vi "AC Transport Configure.vi"(0 "6221 Address":string="13", 1 "SR860 Ch1 Address":string="4", 2 "Ch1 Enable":bool=TRUE, 3 "SR860 Ch2 Address":string="5", 4 "Ch2 Enable":bool=TRUE, 5 "Current Amplitude":string="1e-4", 7 "Frequency":string="17.32", 9 "Filter BW":T2(ring)=enum."100ms", 11 "Buffer Size (kB)":i32=2, 12 "Ch1 Harmonic":T1(ring), 13 "Ch2 Harmonic":T1(ring), 14 "Rate decimation":i32=2) -> (8 "Error 6221":errorcluster, 10 "Error SR860 Ch1":errorcluster, 15 "Error SR860 Ch2":errorcluster)   [LabVIEW 2020]
panel:
  in  "INIT 6221":bool=TRUE
  in  "Buffer Data":enum16{"X", "XY", "RT", "XYRT"}(ring)=enum."RT"
  out "SR860 Commands":string="*RST;\nIVMD VOLTAGE;\nISRC A-B;\nICPL AC;\nIGND GROund;\nSYNC OFF;\nOFSL 3;\nOFLT 10;\nRSRC EXT;\nRTRG NEGttl;\nREFZ 1Meg;\nHARM 1;\nARNG;\nASCL;\nAPHS;\nCAPTURELEN 2;\nCAPTURECFG 2;\nCAPTURERATE 2;\n"
  in  "TRIG Wave":bool
  out "6221 Commands":string="*RST\nTRIG:OLIN 4\nOUTP:LTEarth ON\nSOUR:WAVE:AMPL 1e-4\nSOUR:WAVE:FREQ 17.32\nSOUR:WAVE:FUNC SIN\nSOUR:WAVE:OFFS 0\nSOUR:WAVE:PMAR:STAT ON\nSOUR:WAVE:PMAR:OLIN 2\nSOUR:WAVE:RANG BEST\nSOUR:CURR:COMP 25\nSOUR:WAVE:ARM"
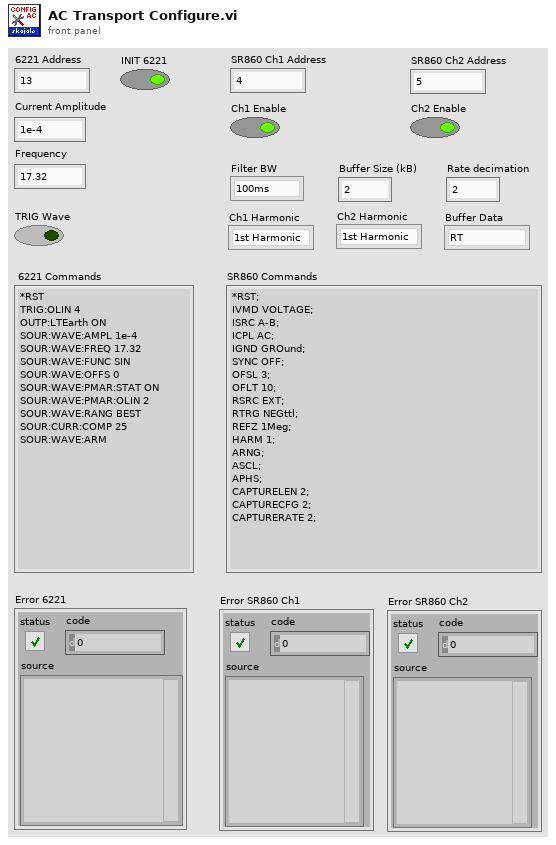
[diagram p1: front panel]
types:
  T1 = enum16{"1st Harmonic", "2nd Harmonic", "3rd Harmonic"}
  T2 = enum16{"1us", "3us", "10us", "30us", "100us", "300us", "1ms", "3ms", "10ms", "30ms", "100ms", "300ms", "1s"}
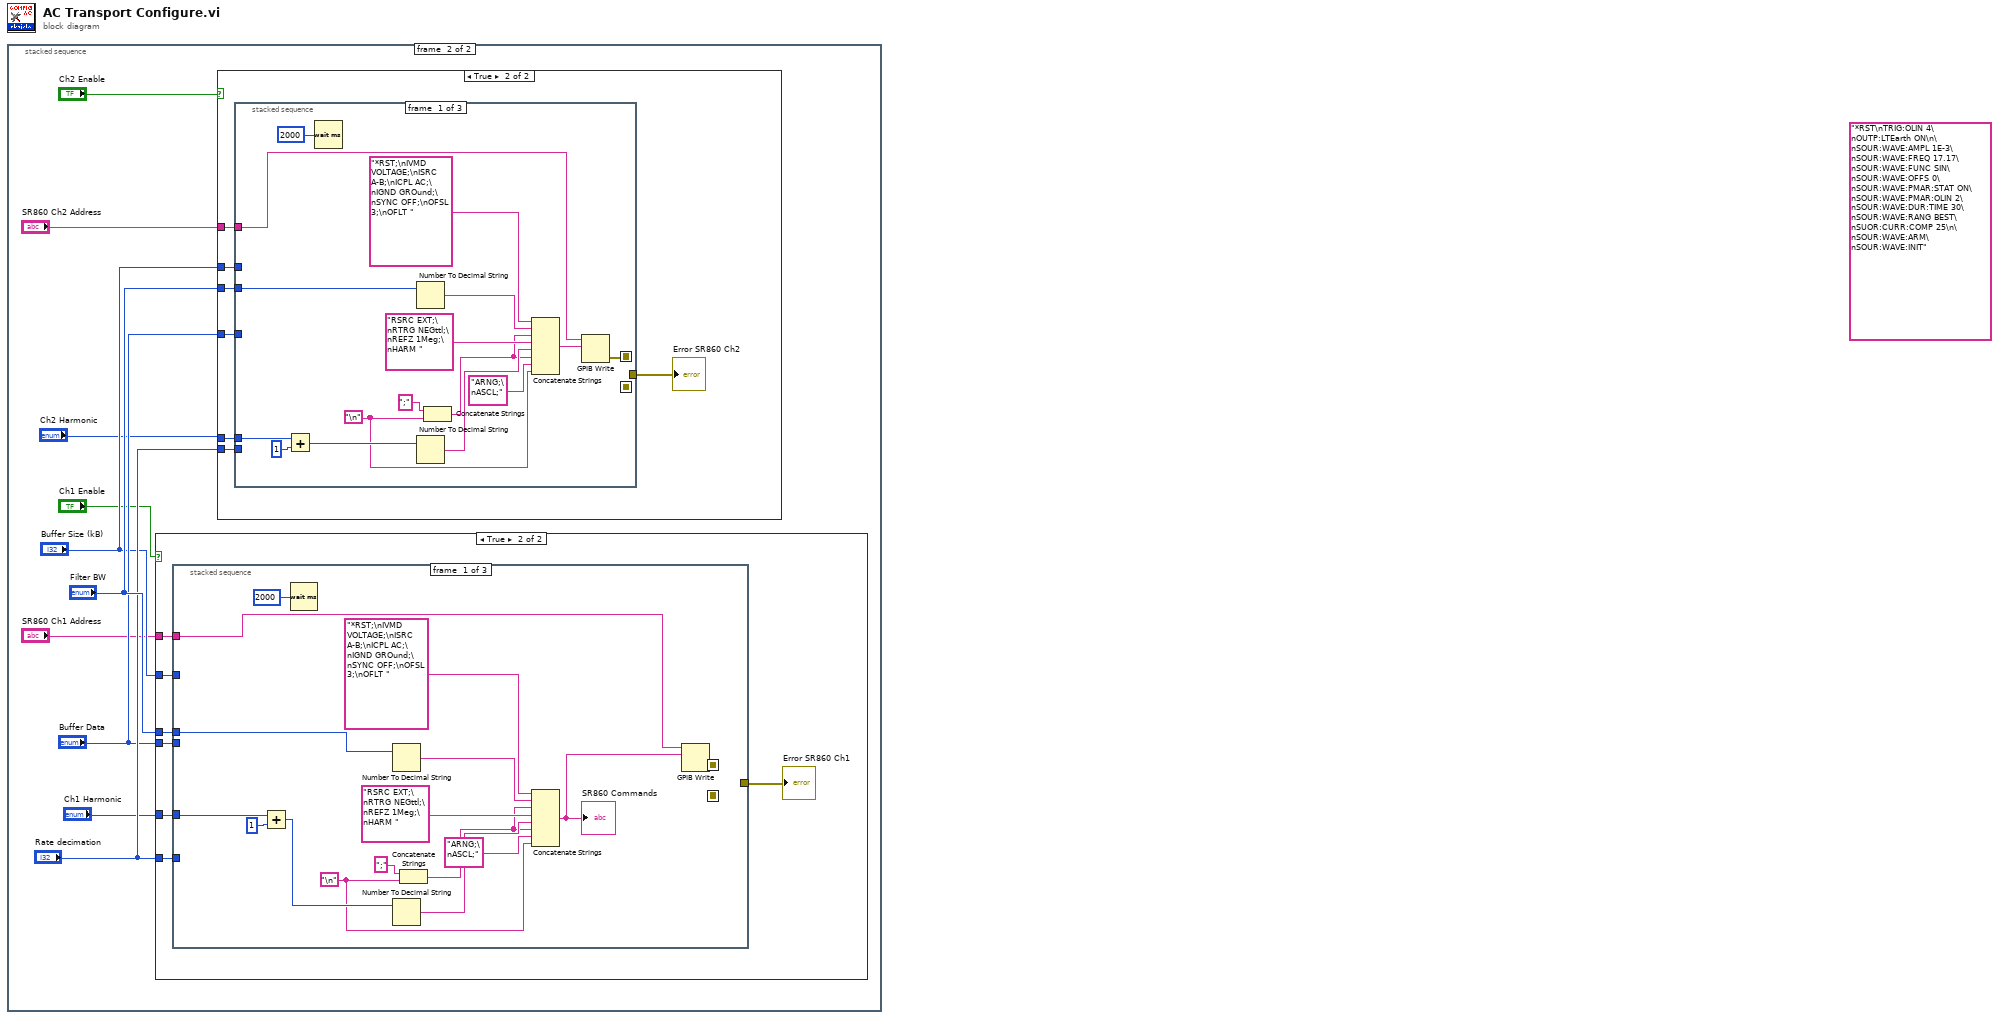
[diagram p0: block diagram]
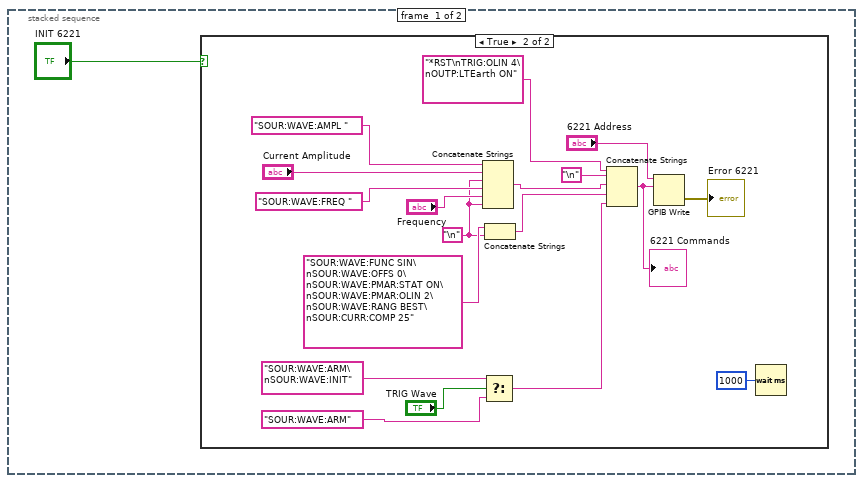
[diagram p2: hidden frame]
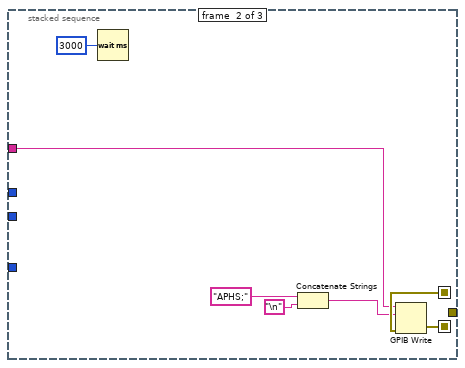
[diagram p5: hidden frame]
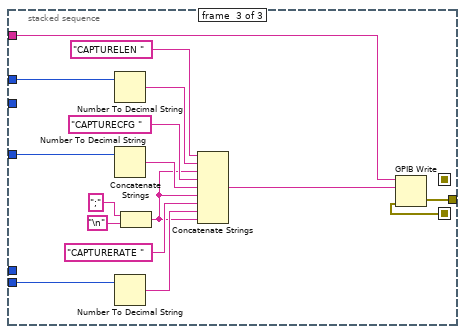
[diagram p6: hidden frame]
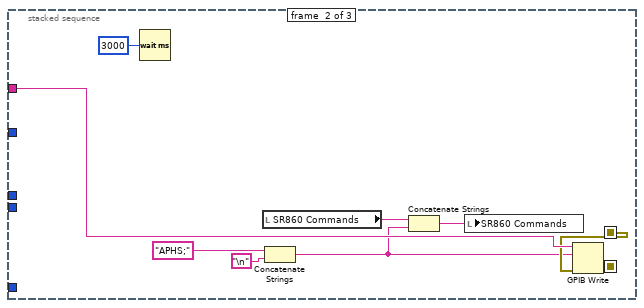
[diagram p8: hidden frame]
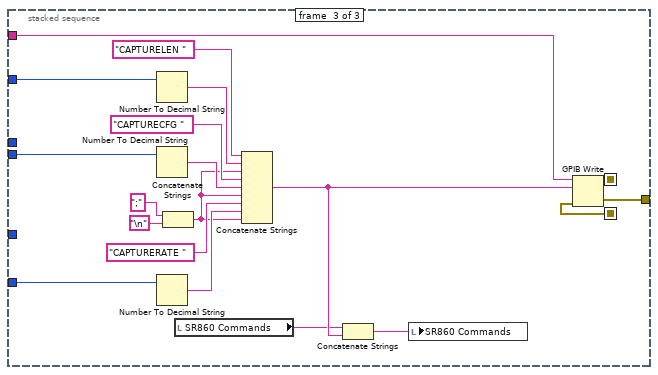
[diagram p9: hidden frame]
diagram:
  (unwired) "*RST\nTRIG:OLIN 4\nOUTP:LTEarth ON\n\nSOUR:WAVE:AMPL 1E-3\nSOUR:WAVE:FREQ 17.17\nSOUR:WAVE:FUNC SIN\nSOUR:WAVE:OFFS 0\nSOUR:WAVE:PMAR:STAT ON\nSOUR:WAVE:PMAR:OLIN 2\nSOUR:WAVE:DUR:TIME 30\nSOUR:WAVE:RANG BEST\nSUOR:CURR:COMP 25\n\nSOUR:WAVE:ARM\nSOUR:WAVE:INIT" ("data")
  n1 = stacked-sequence {
    frame #0 {
      n2 = case shown="True" "INIT 6221" {
        frame False {
        }
        frame True {
          w4 = "\n"
          n3 = Concatenate Strings("SOUR:WAVE:AMPL ", "Current Amplitude", w4, "SOUR:WAVE:FREQ ", "Frequency", w4) -> (w14:string)
          n4 = Select(t="SOUR:WAVE:ARM\nSOUR:WAVE:INIT" ("string"), s="TRIG Wave", f="SOUR:WAVE:ARM" ("string")) -> (s? t:f=w10:string)
          n5 = Concatenate Strings("SOUR:WAVE:FUNC SIN\nSOUR:WAVE:OFFS 0\nSOUR:WAVE:PMAR:STAT ON\nSOUR:WAVE:PMAR:OLIN 2\nSOUR:WAVE:RANG BEST\nSOUR:CURR:COMP 25", w4) -> (w13:string)
          n6 = Concatenate Strings("*RST\nTRIG:OLIN 4\nOUTP:LTEarth ON", "\n", w14, w13, w10) -> (w12:string)
          "6221 Commands" <- w12
          n7 = GPIB Write(0:"6221 Address", 1:w12) -> (6:→"Error 6221":errorcluster)  [unwired: 3 in, 1 out]
          n8 = Wait (ms)(milliseconds to wait=u32 1000) -> ()  [unwired: 1 out]
        }
      }
    }
    frame #1 {
      n9 = case shown="True" "Ch1 Enable" {
        tunnel: "SR860 Ch1 Address" -> [_ w82]
        tunnel: "Rate decimation" -> [_ w80]
        tunnel: "Buffer Data" -> [_ w79]
        tunnel: "Buffer Size (kB)" -> [_ w78]
        tunnel: "Filter BW" -> [_ w77]
        tunnel: "Ch1 Harmonic" -> [_ w76]
        frame False {
        }
        frame True {
          n10 = stacked-sequence {
            seq-local: [w85 _ _] -> [_ w106 _]
            seq-local: [_ w105 _] -> [_ _ w116]
            tunnel: w82 -> [w86 w107 w114]
            tunnel: [_ _ w115] -> w81
            tunnel: w80 -> [_ _ w110]
            tunnel: w79 -> [_ _ w109]
            tunnel: w78 -> [_ _ w108]
            tunnel: w77 -> [w84 _ _]
            tunnel: w76 -> [w83 _ _]
            frame #0 {
              w89 = "\n"
              n11 = Add(x=w83, y=1) -> (x+y=w92:i32)
              n12 = Wait (ms)(milliseconds to wait=u32 2000) -> ()  [unwired: 1 out]
              n13 = Number To Decimal String(number=w84) -> (decimal integer string=w97:string)  [unwired: 1 in]
              n14 = Number To Decimal String(number=w92) -> (decimal integer string=w94:string)  [unwired: 1 in]
              n15 = Concatenate Strings(";" ("string"), w89) -> (w93:string)
              n16 = Concatenate Strings("*RST;\nIVMD VOLTAGE;\nISRC A-B;\nICPL AC;\nIGND GROund;\nSYNC OFF;\nOFSL 3;\nOFLT ", w97, w93, "RSRC EXT;\nRTRG NEGttl;\nREFZ 1Meg;\nHARM ", w94, w93, "ARNG;\nASCL;", w89) -> (w87:string)
              "SR860 Commands" <- w87
              n17 = GPIB Write(0:w86, 1:w87) -> (6:w85:errorcluster)  [unwired: 3 in, 1 out]
            }
            frame #1 {
              n18 = Wait (ms)(milliseconds to wait=u32 3000) -> ()  [unwired: 1 out]
              n19 = local read "SR860 Commands"() -> (w101:string)
              n20 = Concatenate Strings("APHS;", "\n") -> (w102:string)
              n21 = Concatenate Strings(w101, w102) -> (w100:string)
              n22 = local write "SR860 Commands"(w100) -> ()
              n23 = GPIB Write(0:w107, 1:w102, 3:w106) -> (6:w105:errorcluster)  [unwired: 2 in, 1 out]
            }
            frame #2 {
              n24 = Number To Decimal String(number=w108) -> (decimal integer string=w124:string)  [unwired: 1 in]
              n25 = Number To Decimal String(number=w109) -> (decimal integer string=w121:string)  [unwired: 1 in]
              n26 = Number To Decimal String(number=w110) -> (decimal integer string=w118:string)  [unwired: 1 in]
              n27 = Concatenate Strings(";" ("string"), "\n") -> (w117:string)
              n28 = local read "SR860 Commands"() -> (w111:string)
              n29 = Concatenate Strings("CAPTURELEN ", w124, w117, "CAPTURECFG ", w121, w117, "CAPTURERATE ", w118, w117) -> (w113:string)
              n30 = Concatenate Strings(w111, w113) -> (w112:string)
              n31 = local write "SR860 Commands"(w112) -> ()
              n32 = GPIB Write(0:w114, 1:w113, 3:w116) -> (6:w115:errorcluster)  [unwired: 2 in, 1 out]
            }
          }
          "Error SR860 Ch1" <- w81
        }
      }
      n33 = case shown="True" "Ch2 Enable" {
        tunnel: "Buffer Size (kB)" -> [_ w35]
        tunnel: "Buffer Data" -> [_ w34]
        tunnel: "Rate decimation" -> [_ w33]
        tunnel: "Filter BW" -> [_ w32]
        tunnel: "Ch2 Harmonic" -> [_ w31]
        tunnel: "SR860 Ch2 Address" -> [_ w30]
        frame False {
        }
        frame True {
          n34 = stacked-sequence {
            seq-local: [w40 _ _] -> [_ w59 _]
            seq-local: [_ w58 _] -> [_ _ w66]
            tunnel: [_ _ w65] -> w36
            tunnel: w35 -> [_ _ w63]
            tunnel: w34 -> [_ _ w62]
            tunnel: w33 -> [_ _ w61]
            tunnel: w32 -> [w39 _ _]
            tunnel: w31 -> [w38 _ _]
            tunnel: w30 -> [w37 w53 w60]
            frame #0 {
              w43 = "\n"
              n35 = Add(x=w38, y=1) -> (x+y=w46:i32)
              n36 = Wait (ms)(milliseconds to wait=u32 2000) -> ()  [unwired: 1 out]
              n37 = Number To Decimal String(number=w39) -> (decimal integer string=w51:string)  [unwired: 1 in]
              n38 = Number To Decimal String(number=w46) -> (decimal integer string=w48:string)  [unwired: 1 in]
              n39 = Concatenate Strings(";" ("string"), w43) -> (w47:string)
              n40 = Concatenate Strings("*RST;\nIVMD VOLTAGE;\nISRC A-B;\nICPL AC;\nIGND GROund;\nSYNC OFF;\nOFSL 3;\nOFLT ", w51, w47, "RSRC EXT;\nRTRG NEGttl;\nREFZ 1Meg;\nHARM ", w48, w47, "ARNG;\nASCL;", w43) -> (w41:string)
              n41 = GPIB Write(0:w37, 1:w41) -> (6:w40:errorcluster)  [unwired: 3 in, 1 out]
            }
            frame #1 {
              n42 = Wait (ms)(milliseconds to wait=u32 3000) -> ()  [unwired: 1 out]
              n43 = Concatenate Strings("APHS;", "\n") -> (w55:string)
              n44 = GPIB Write(0:w53, 1:w55, 3:w59) -> (6:w58:errorcluster)  [unwired: 2 in, 1 out]
            }
            frame #2 {
              n45 = Number To Decimal String(number=w63) -> (decimal integer string=w74:string)  [unwired: 1 in]
              n46 = Number To Decimal String(number=w62) -> (decimal integer string=w71:string)  [unwired: 1 in]
              n47 = Number To Decimal String(number=w61) -> (decimal integer string=w68:string)  [unwired: 1 in]
              n48 = Concatenate Strings(";" ("string"), "\n") -> (w67:string)
              n49 = Concatenate Strings("CAPTURELEN ", w74, w67, "CAPTURECFG ", w71, w67, "CAPTURERATE ", w68, w67) -> (w64:string)
              n50 = GPIB Write(0:w60, 1:w64, 3:w66) -> (6:w65:errorcluster)  [unwired: 2 in, 1 out]
            }
          }
          "Error SR860 Ch2" <- w36
        }
      }
    }
  }
